vi "Encoder.vi"(11 "Reset Counter":bool) -> (2 "Counter Direction":T1, 3 "Counter Value":i32)   [LabVIEW 2017]
uses:
  <vilib>/myRIO/Common/Instrument Driver Framework/myRIO v1.0/Encoder/typedefs/Encoder Count Direction Enum.ctl
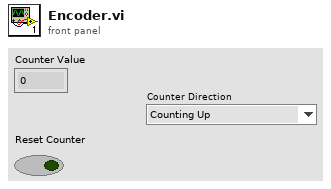
[diagram p1: front panel]
types:
  T1 = typedef "Encoder Count Direction Enum.ctl" = enum16{"Counting Up", "Counting Down"}
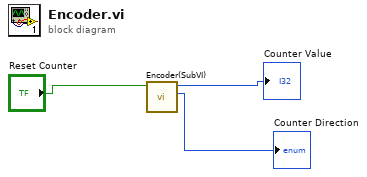
[diagram p0: block diagram]
diagram:
  n1 = call "Encoder(SubVI).vi"("Reset Counter"="Reset Counter") -> ("Counter Direction"=→"Counter Direction":T1, "Counter Value"=→"Counter Value":i32)  [unwired: 9 in]
